vi "Read Tags.vi"(8 "error in (no error)":errorcluster, 11 "Var_Access in":refnum<class "Var_Access.lvclass">) -> (0 "error out":errorcluster, 2 "Tags":string[](array[string]), 3 "Var_Access out":refnum<class "Var_Access.lvclass">)   [LabVIEW 2021, in "Var_Access.lvclass"]
uses:
  Var_Access.lvclass
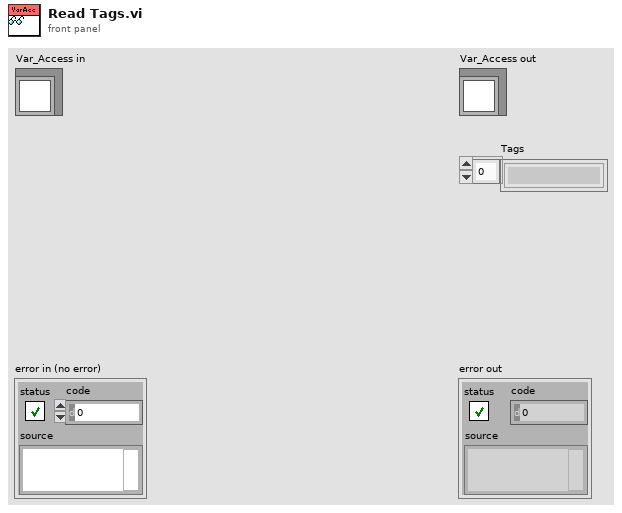
[diagram p1: front panel]
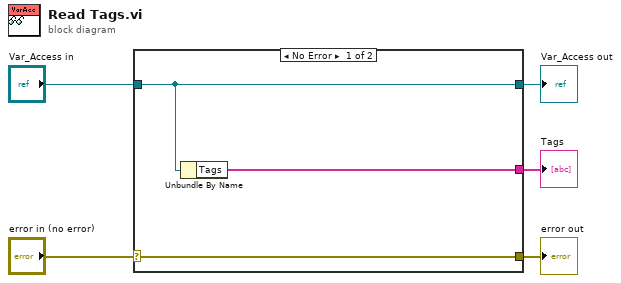
[diagram p0: block diagram]
diagram:
  n1 = case shown="No Error" "error in (no error)" {
    selector: "error in (no error)" -> [w8 w9]
    tunnel: [w8 w9] -> w4
    tunnel: [w7 w10] -> w2
    tunnel: "Var_Access in" -> [w7 w10]
    tunnel: [w6 _] -> w1
    frame No Error {
      n2 = Unbundle By Name(w7) -> ("Tags"=w6:string[])
    }
    frame Error {
    }
  }
  "error out" <- w4
  "Var_Access out" <- w2
  "Tags" <- w1
